vi "Debug Values.vi"(8 "error in (no error)":errorcluster, 11 "Session in":refnum<class "Session.lvclass">) -> (0 "error out":errorcluster, 2 "Session Debug Info":T1, 3 "Session out":refnum<class "Session.lvclass">)   [LabVIEW 2020, in "HTTP Server.lvlib" / "Session.lvclass"]
uses:
  Session.lvclass
  Session Debug Info.ctl
  Session.lvclass/Session.ctl
  HTTP Server.lvlib
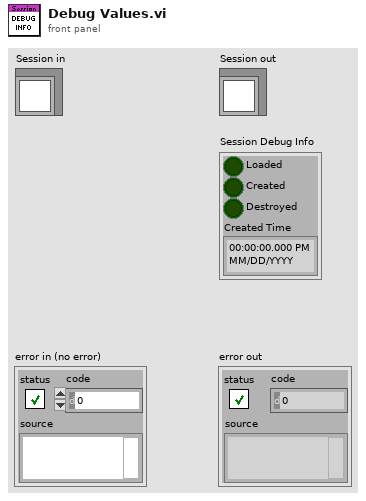
[diagram p1: front panel]
types:
  T1 = typedef "HTTP Server.lvlib/Session Debug Info.ctl" = cluster{"Loaded":bool, "Created":bool, "Destroyed":bool, "Created Time":timestamp}
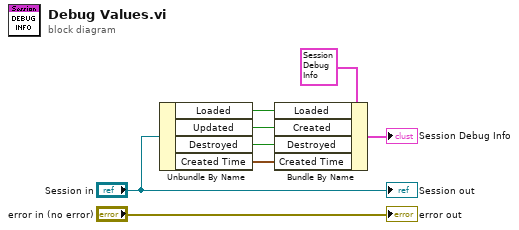
[diagram p0: block diagram]
diagram:
  n1 = Unbundle By Name("Session in") -> ("Loaded"=w4:bool, "Updated"=w3:bool, "Destroyed"=w2:bool, "Created Time"=w1:timestamp)
  n2 = Bundle By Name(cluster=T1 {"Loaded"=FALSE, "Created"=FALSE, "Destroyed"=FALSE, "Created Time"=timestamp(0 s since 1904-01-01)} ("Session Debug Info"), "Loaded"=w4, "Created"=w3, "Destroyed"=w2, "Created Time"=w1) -> (→"Session Debug Info":T1)
  "error out" <- "error in (no error)"
  "Session out" <- "Session in"
